vi "Set Pod Setpoints.vi"(8 "Steer Angles (ticks)":T1, 9 "Drive Velocities (ticks/ds)":T1, 10 "Pod Setpoints (ft/s and deg)":T10, 11 "Motors":T3) -> ()   [LabVIEW 2020]
uses:
  ctl/Pod Setpoints.ctl
  ctl/Swerve Motors.ctl
  ctl/4 Motor Set.ctl
  <vilib>/Rock Robotics/WPI/MotorControl/WPI_MotorControlDeviceRef.ctl
  <vilib>/Rock Robotics/WPI/MotorControl/WPI_MotorControlType.ctl
  <vilib>/Rock Robotics/SystemInterfaces/DIO/FPGA_DIOPWMChannel.ctl
  <vilib>/Rock Robotics/WPI/PWM/WPI_PWMDeadband.ctl
  <vilib>/Rock Robotics/SystemInterfaces/DIO/FPGA_DIOChannel.ctl
  <vilib>/Rock Robotics/WPI/ThirdParty/Phoenix-LabVIEW/Motor Controller/Controls/CTRE_Phoenix_MotorControl_ControlMode.ctl
  dae1c354-363e-4ff0-b5a6-c321b13c3a50.vi
panel:
  in  "Push PID":bool
  out "PID Graph":cluster{"Left Front":i32, "Theta":dbl}(graph)
  in  "PID Coefficients":cluster{"P":dbl, "I":dbl, "D":dbl, "F":dbl}
  in  "Motor Position":T2(ring)
  in  "Motor Type":enum16{"Drive", "Steer"}(ring)
  in  "Debug Mode?":bool
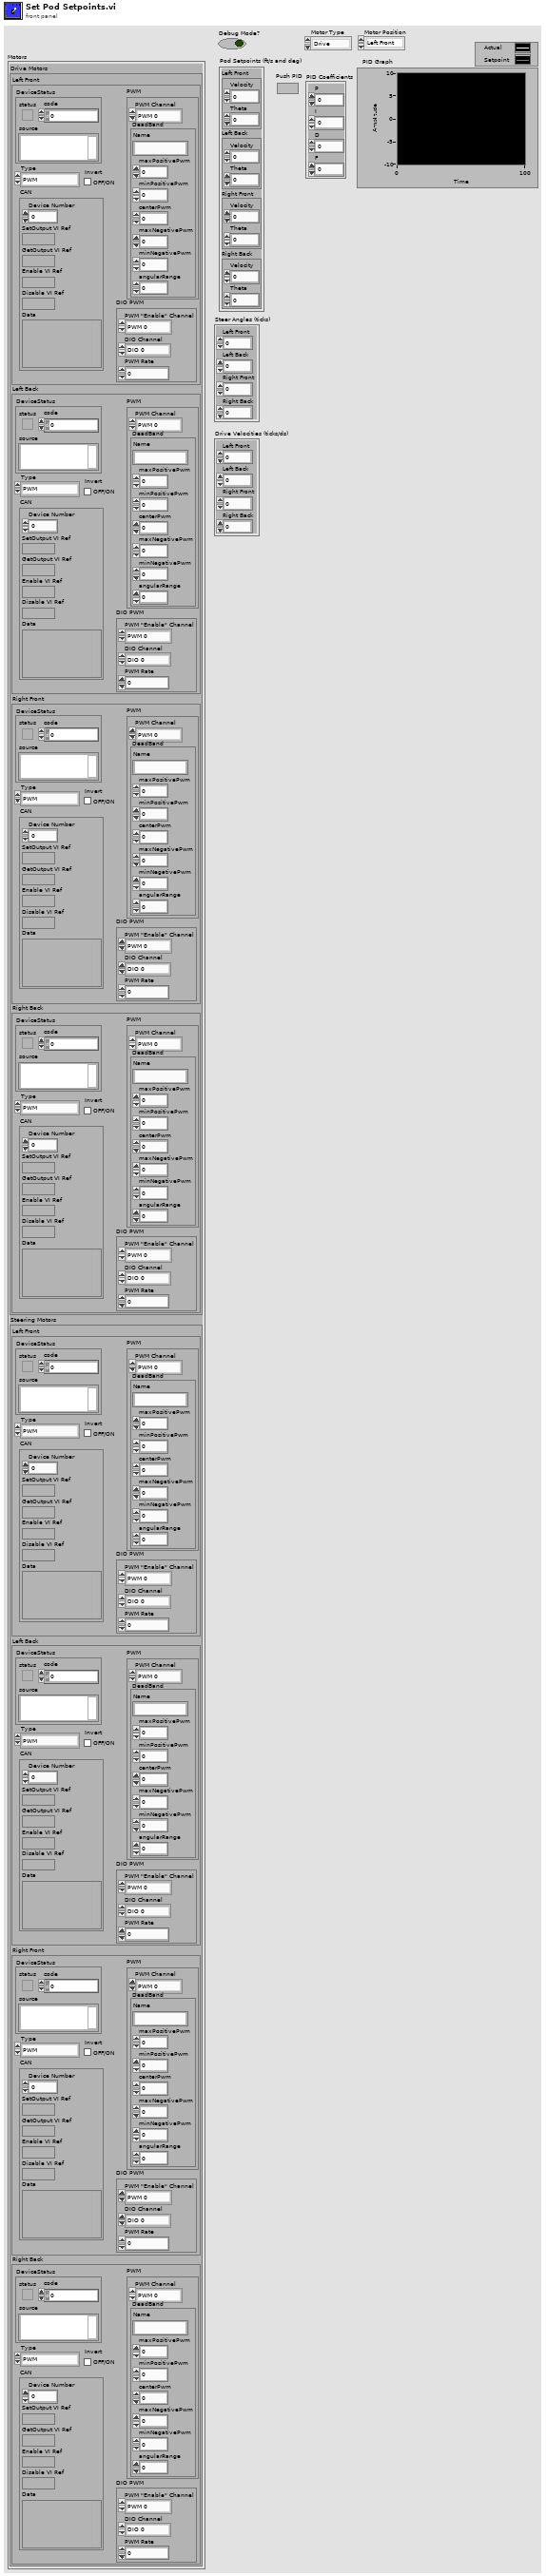
[diagram p1: front panel]
types:
  T1 = cluster{"Left Front":i32, "Left Back":i32, "Right Front":i32, "Right Back":i32}
  T2 = enum16{"Left Front", "Left Back", "Right Front", "Right Back"}
  T3 = typedef "Swerve Motors.ctl" = cluster{"Drive Motors":T4, "Steering Motors":T4}
  T4 = typedef "4 Motor Set.ctl" = cluster{"Left Front":T5, "Left Back":T5, "Right Front":T5, "Right Back":T5}
  T5 = typedef "WPI_MotorControlDeviceRef.ctl" = cluster{"DeviceStatus":errorcluster, "Type":T6, "PWM":cluster{"PWM Channel":T7, "DeadBand":T8}, "CAN":cluster{"Device Number":u8, "SetOutput VI Ref":variant, "GetOutput VI Ref":variant, "Enable VI Ref":variant, "Disable VI Ref":variant, "Data":variant}, "Invert":bool, "DIO PWM":cluster{"PWM \"Enable\" Channel":T7, "DIOChannel":T9, "PWM Rate":dbl}}
  T6 = typedef "WPI_MotorControlType.ctl" = enum16{"PWM", "CAN", "DIO PWM"}
  T7 = typedef "FPGA_DIOPWMChannel.ctl" = enum8{"PWM 0", "PWM 1", "PWM 2", "PWM 3", "PWM 4", "PWM 5", "PWM 6", "PWM 7", "PWM 8", "PWM 9", "PWM MXP 0", "PWM MXP 1", "PWM MXP 2", "PWM MXP 3", "PWM MXP 4", "PWM MXP 5", "PWM MXP 6", "PWM MXP 7", "PWM MXP 8", "PWM MXP 9", "Invalid"}
  T8 = typedef "WPI_PWMDeadband.ctl" = cluster{"Name":string, "maxPositivePwm":i32, "minPositivePwm":i32, "centerPwm":i32, "maxNegativePwm":i32, "minNegativePwm":i32, "angularRange":u16}
  T9 = typedef "FPGA_DIOChannel.ctl" = enum8{"DIO 0", "DIO 1", "DIO 2", "DIO 3", "DIO 4", "DIO 5", "DIO 6", "DIO 7", "DIO 8", "DIO 9", "DIO MXP 0", "DIO MXP 1", "DIO MXP 2", "DIO MXP 3", "DIO MXP 4", "DIO MXP 5", "DIO MXP 6", "DIO MXP 7", "DIO MXP 8", "DIO MXP 9", "DIO MXP 10", "DIO MXP 11", "DIO MXP 12", "DIO MXP 13", "DIO MXP 14", "DIO MXP 15", "SPI Port CS1", "SPI Port CS2", "SPI Port CS3", "SPI Port MISO", "SPI Port MOSI", "Invalid"}
  T10 = typedef "Pod Setpoints.ctl" = cluster{"Left Front":cluster{"Velocity":dbl, "Theta":dbl}, "Left Back":cluster{"Velocity":dbl, "Theta":dbl}, "Right Front":cluster{"Velocity":dbl, "Theta":dbl}, "Right Back":cluster{"Velocity":dbl, "Theta":dbl}}
  T11 = typedef "CTRE_Phoenix_MotorControl_ControlMode.ctl" = u16
  T12 = cluster{"[0]":dbl, "[1]":dbl, "[2]":dbl, "[3]":dbl}
  T13 = cluster{"Left Front":dbl, "Left Back":dbl, "Right Front":dbl, "Right Back":dbl}
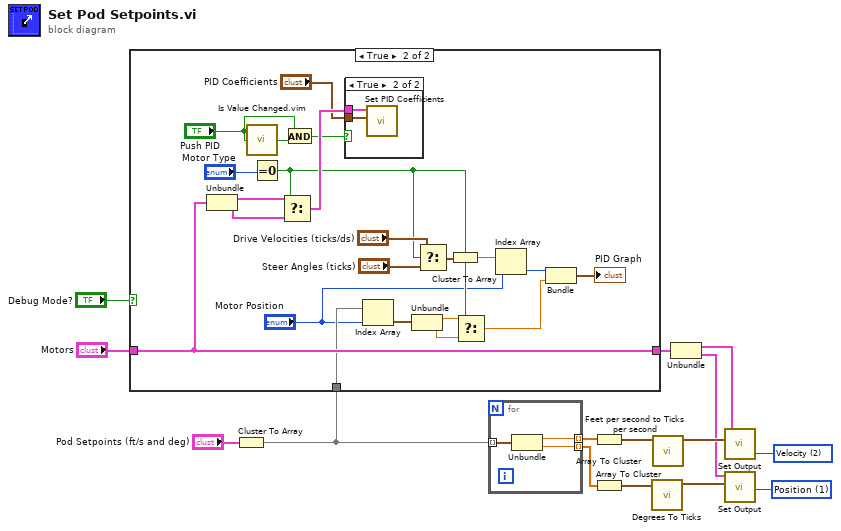
[diagram p0: block diagram]
diagram:
  w4 = T11 1 items=["PercentOutput"=0, "Position"=1, "Velocity"=2, "Current"=3, "Follower"=5, "MotionProfile"=6, "MotionMagic"=7, "MotionProfileArc"=10, "Disabled"=15] ("Control Mode")
  w5 = T11 2 items=["PercentOutput"=0, "Position"=1, "Velocity"=2, "Current"=3, "Follower"=5, "MotionProfile"=6, "MotionMagic"=7, "MotionProfileArc"=10, "Disabled"=15] ("Control Mode")
  n1 = Cluster To Array(cluster="Pod Setpoints (ft/s and deg)") -> (array=w1:cluster{"Velocity":dbl, "Theta":dbl}[])
  n2 = case shown="True" "Debug Mode?" {
    tunnel: "Motors" -> [w16 w38]
    tunnel: [w16 w38] -> w9
    tunnel: w1 -> [_ w34]
    frame False {
    }
    frame True {
      n3 = Unbundle(w38) -> ("Drive Motors"=w36:T4, "Steering Motors"=w35:T4)
      n4 = call "Is Value Changed.vim"("value"="Push PID") -> ("changed or first call?"=w26:bool)
      n5 = Equal To 0?(x="Motor Type") -> (x = 0?=w21:bool)
      n6 = Select(t=w36, s=w21, f=w35) -> (s? t:f=w30:T4)
      n7 = And(x="Push PID", y=w26) -> (x .and. y?=w25:bool)
      n8 = case shown="True" w25 {
        tunnel: w30 -> [_ w40]
        tunnel: "PID Coefficients" -> [_ w39]
        frame False {
        }
        frame True {
          n9 = call "Set PID Coefficients.vi"("PID Coefficients"=w39, "Motors"=w40) -> ()  [unwired: 10 in]
        }
      }
      n10 = Index Array(array=w34, index="Motor Position") -> (element=w33:cluster{"Velocity":dbl, "Theta":dbl})
      n11 = Unbundle(w33) -> ("Velocity"=w32:dbl, "Theta"=w31:dbl)
      n12 = Select(t="Drive Velocities (ticks/ds)", s=w21, f="Steer Angles (ticks)") -> (s? t:f=w20:T1)
      n13 = Cluster To Array(cluster=w20) -> (array=w19:i32[])
      n14 = Select(t=w32, s=w21, f=w31) -> (s? t:f=w29:dbl)
      n15 = Index Array(array=w19, index="Motor Position") -> (element=w17:i32)
      n16 = Bundle("Left Front"=w17, "Theta"=w29) -> (→"PID Graph":cluster{"Left Front":i32, "Theta":dbl})  [unwired: 1 in]
    }
  }
  n17 = for {
    tunnel: w1 -> [w43] mode=indexing
    tunnel: [w42] -> w15 mode=indexing
    tunnel: [w41] -> w14 mode=indexing
    n18 = Unbundle(w43) -> ("Velocity"=w42:dbl, "Theta"=w41:dbl)
  }
  n19 = Array To Cluster(array=w15) -> (cluster=w12:T12)
  n20 = Array To Cluster(array=w14) -> (cluster=w13:T12)
  n21 = call "Degrees To Ticks.vi"("Steering Angles (degrees)"=w13) -> ("Steering Angles (ticks)"=w7:T13)  [unwired: 10 in]
  n22 = call "Feet per second to Ticks per second.vi"("Drive Velocities (ft/s)"=w12) -> ("Drive Velocities (ticks/ds)"=w6:T13)  [unwired: 10 in]
  n23 = Unbundle(w9) -> ("Drive Motors"=w8:T4, "Steering Motors"=w3:T4)
  n24 = call "Set Output.vi"("Control Mode"=w5, "Setpoints"=w6, "Motors"=w8) -> ()  [unwired: 9 in]
  n25 = call "Set Output.vi"("Control Mode"=w4, "Setpoints"=w7, "Motors"=w3) -> ()  [unwired: 9 in]
